vi "ForceProgram.vi"() -> ()   [LabVIEW 2014]
uses:
  <vilib>/express/express shared/transition.llb/Dynamic To Waveform Array.vi
  <vilib>/express/express arith-compare/Formula/Block/exnFormulaBlock how many pts in the wave.vi
  <vilib>/express/express shared/ex_Modify Signal Name.vi
  <vilib>/express/express shared/transition.llb/Waveform Array To Dynamic.vi
  <vilib>/Waveform/WDTOps.llb/WDT Align Waveform Timestamps DBL.vi
  <vilib>/express/express arith-compare/Formula/XNode/ExpressFormulaBlockNode.xnode
panel:
  out "Adjusted Force":dbl
  in  "Manual Offest Adjust":dbl
  out "Baseline (Offset)":dbl
  in  "Radio Buttons 2":T1(radio)
  in  "Specify Output File:":path=path "C:/Users/joe/Documents/LabVIEW Data/Temp/Testname_TestNumber_TestDate.lvm"
  out "Current Force":waveform(dbl)[](graph)
  in  "Exit Program":bool
  in  "Estimated MVC (N)":dbl=150.0
  in  "Dorsi / Plantar":bool
  out "Elapsed Time (s)":dbl format="%#_4g"
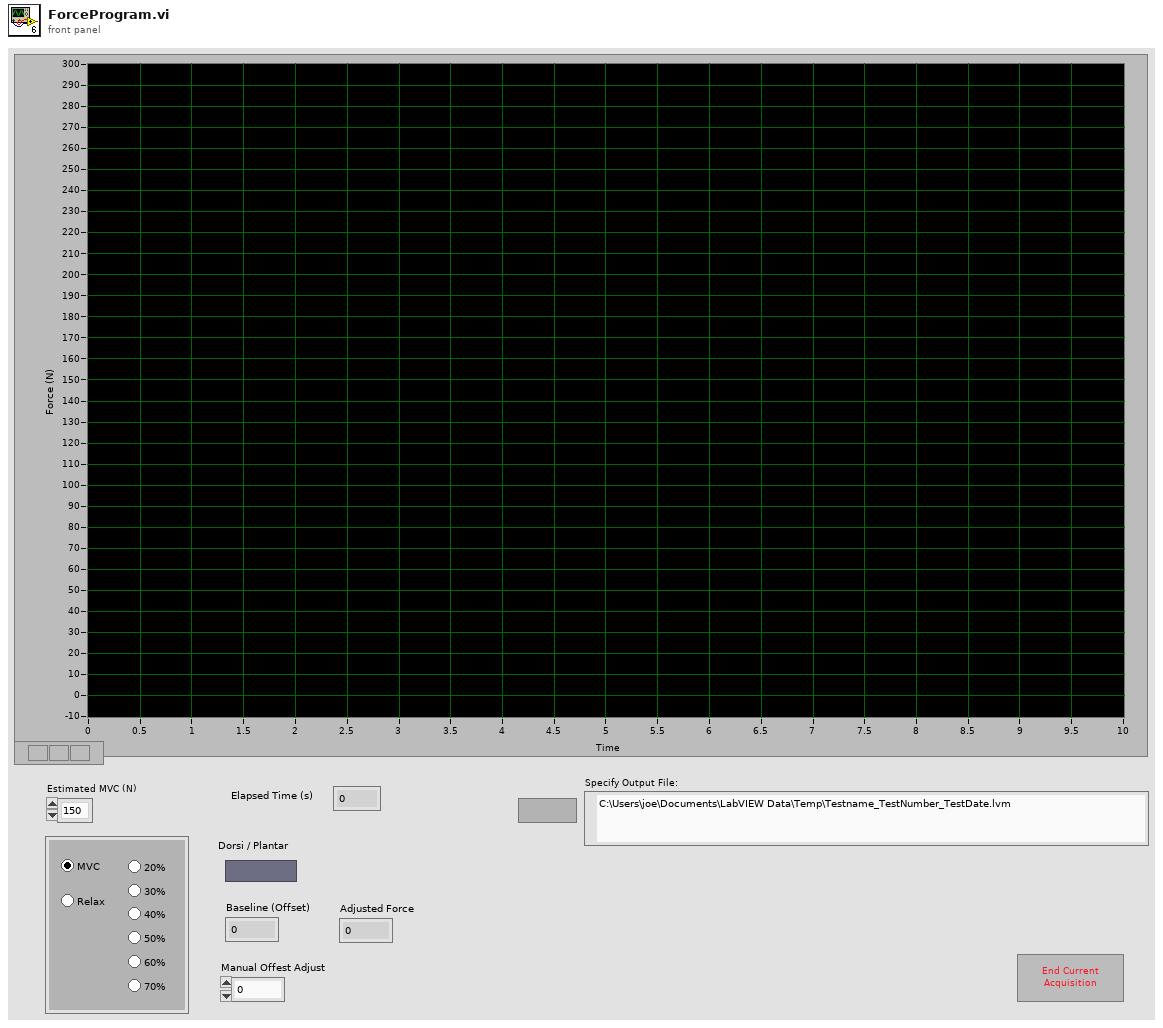
[diagram p1: front panel]
types:
  T1 = enum32{"MVC", "Relax", "20%", "30%", "40%", "50%", "60%", "70%"}
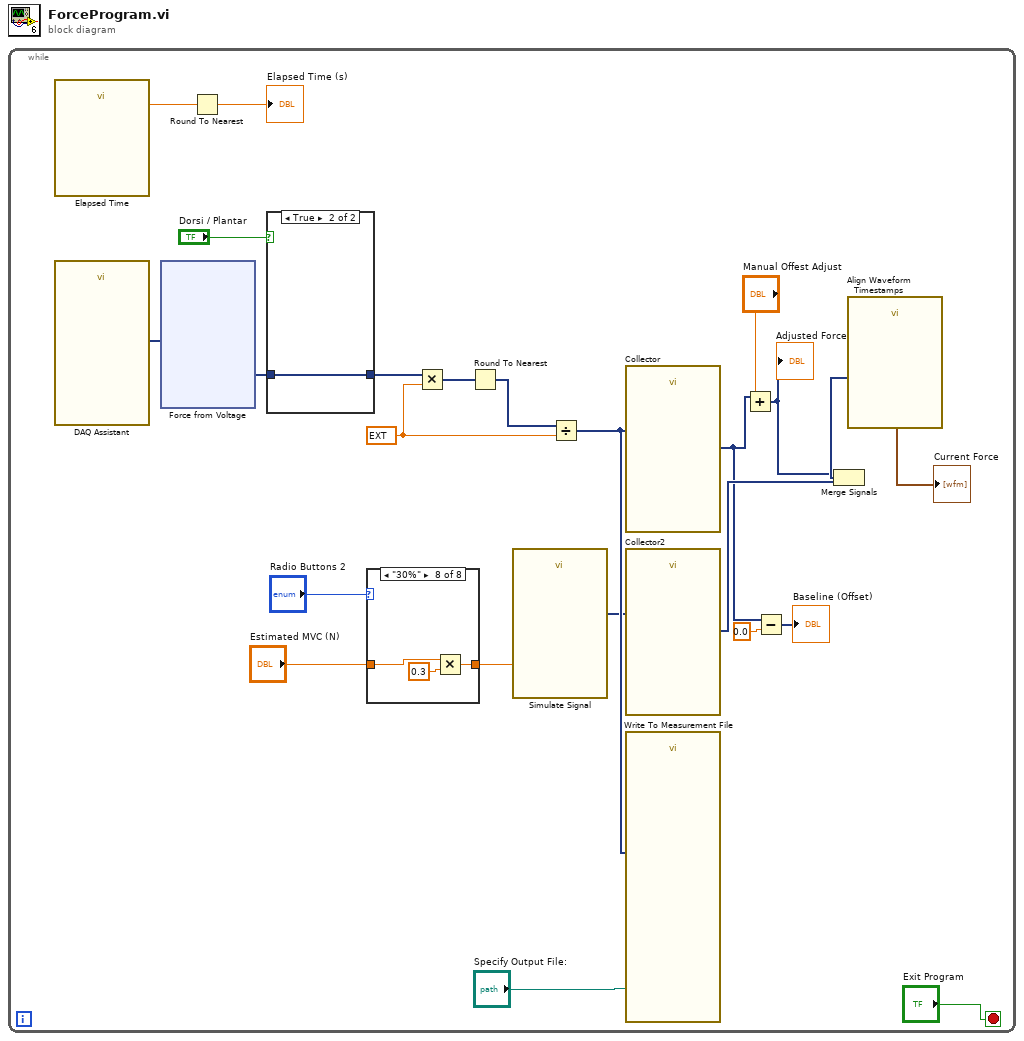
[diagram p0: block diagram]
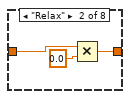
[diagram p3: hidden frame]
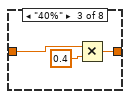
[diagram p4: hidden frame]
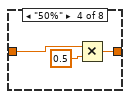
[diagram p5: hidden frame]
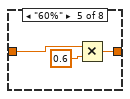
[diagram p6: hidden frame]
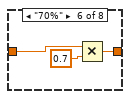
[diagram p7: hidden frame]
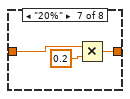
[diagram p8: hidden frame]
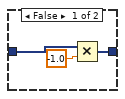
[diagram p9: hidden frame]
diagram:
  n1 = while {
    stop <- "Exit Program" stop-if-true
    w22 = ext 1000.0 ("y")
    n2 = call "Elapsed Time"() -> ("Elapsed Time (s)"=w13:dbl)  [unwired: 12 in, 7 out]
    n3 = call "DAQ Assistant"() -> ("data"=w10:dynamicdata)  [unwired: 16 in, 3 out]
    n4 = xnode "Force from Voltage"("X1"=w10) -> ("Result"=w15:dynamicdata)  [unwired: 1 in, 1 out]
    n5 = Round To Nearest(number=w13) -> (nearest integer value=→"Elapsed Time (s)":dbl)
    n6 = case shown="True" "Dorsi / Plantar" {
      tunnel: w15 -> [w48 w50]
      tunnel: [w47 w50] -> w11
      frame False {
        n7 = Multiply(x=w48, y=-1.0) -> (x*y=w47:dynamicdata)
      }
      frame True {
      }
    }
    n8 = case shown="\"30%\"" "Radio Buttons 2" {
      tunnel: "Estimated MVC (N)" -> [w25 w27 w30 w33 w36 w39 w42 w45]
      tunnel: [w25 w26 w29 w32 w35 w38 w41 w44] -> w7
      frame "MVC", Default {
      }
      frame "Relax" {
        n9 = Multiply(x=w27, y=0.0) -> (x*y=w26:dbl)
      }
      frame "40%" {
        n10 = Multiply(x=w30, y=0.4) -> (x*y=w29:dbl)
      }
      frame "50%" {
        n11 = Multiply(x=w33, y=0.5) -> (x*y=w32:dbl)
      }
      frame "60%" {
        n12 = Multiply(x=w36, y=0.6) -> (x*y=w35:dbl)
      }
      frame "70%" {
        n13 = Multiply(x=w39, y=0.7) -> (x*y=w38:dbl)
      }
      frame "20%" {
        n14 = Multiply(x=w42, y=0.2) -> (x*y=w41:dbl)
      }
      frame "30%" {
        n15 = Multiply(x=w45, y=0.3) -> (x*y=w44:dbl)
      }
    }
    n16 = Multiply(x=w11, y=w22) -> (x*y=w24:dynamicdata)
    n17 = Round To Nearest(number=w24) -> (nearest integer value=w23:dynamicdata)
    n18 = call "Simulate Signal"("Offset"=w7) -> ("DC"=w9:dynamicdata)  [unwired: 13 in, 1 out]
    n19 = Divide(x=w23, y=w22) -> (x/y=w19:dynamicdata)
    n20 = call "Collector"("Signals"=w19) -> ("Collected Signals"=w2:dynamicdata)  [unwired: 9 in, 1 out]
    n21 = call "Collector2"("Signals"=w9) -> ("Collected Signals"=w16:dynamicdata)  [unwired: 9 in, 1 out]
    n22 = call "Write To Measurement File"("Signals"=w19, "Filename"="Specify Output File:") -> ()  [unwired: 15 in, 3 out]
    n23 = Add(x=w2, y="Manual Offest Adjust") -> (x+y=w1:dynamicdata)
    "Adjusted Force" <- w1
    n24 = Subtract(x=w2, y=0.0) -> (x-y=→"Baseline (Offset)":dynamicdata)
    n25 = Merge Signals(w1, w16) -> (w18:dynamicdata)
    n26 = call-poly <vilib>:"Align Waveform Timestamps.vi"("waveforms in"=w18) -> ("waveforms out"=→"Current Force":waveform(dbl)[])  [unwired: 9 in, 1 out]
  }
